vi "unsubscribe_close.vi"(8 "连接ID":refnum<k5>, 11 "topic":string="/chatter") -> ()   [LabVIEW 2014]
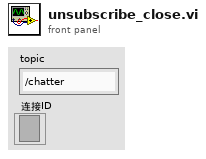
[diagram p1: front panel]
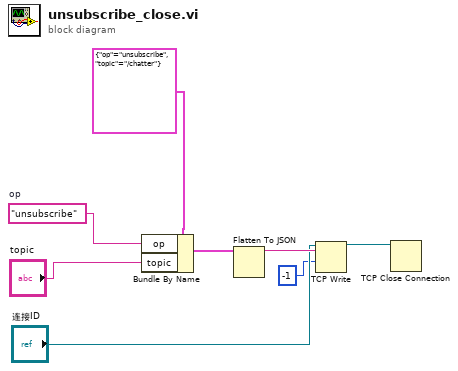
[diagram p0: block diagram]
diagram:
  w7 = "unsubscribe"  # op
  n1 = Bundle By Name(cluster=cluster{"op":string, "topic":string} {"op"="unsubscribe", "topic"="/chatter"}, "op"=w7, "topic"="topic") -> (w5:cluster{"op":string, "topic":string})
  n2 = Flatten To JSON(anything=w5) -> (JSON string=w4:string)  [unwired: 2 in, 1 out]
  n3 = TCP Write(connection ID="连接ID", data in=w4, 9:-1 ("超时毫秒(25000)")) -> (connection ID out=w1:refnum<k5>)  [unwired: 1 in, 2 out]
  n4 = TCP Close Connection(connection ID=w1) -> ()  [unwired: 2 in, 2 out]
